vi "GetSourceAutorange.vi"(7 "SMU":T2, 8 "Error In":errorcluster, 10 "Source Function":T1, 11 "Kiethley 2602 In":refnum<visa-resource-name>) -> (0 "Error Out":errorcluster, 2 "Enabled?":bool, 3 "Keithley 2602 Out":refnum<visa-resource-name>)   [LabVIEW 2012, in "Keithley-2602.lvlib"]
uses:
  Keithley-2602.lvlib
  Controls/SMU.ctl
  Controls/SourceFunction.ctl
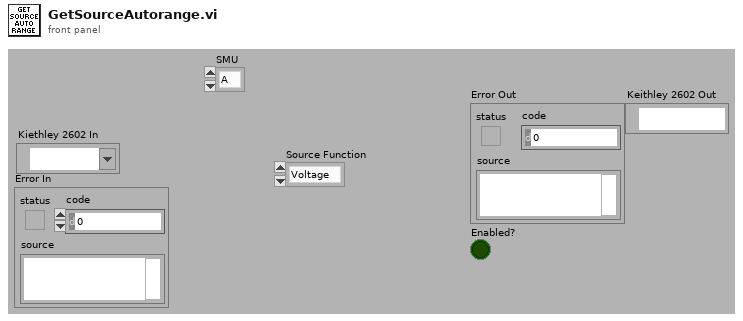
[diagram p1: front panel]
types:
  T1 = typedef "Keithley-2602.lvlib/SourceFunction.ctl" = enum16{"Voltage", "Current"}
  T2 = typedef "Keithley-2602.lvlib/SMU.ctl" = enum16{"A", "B"}
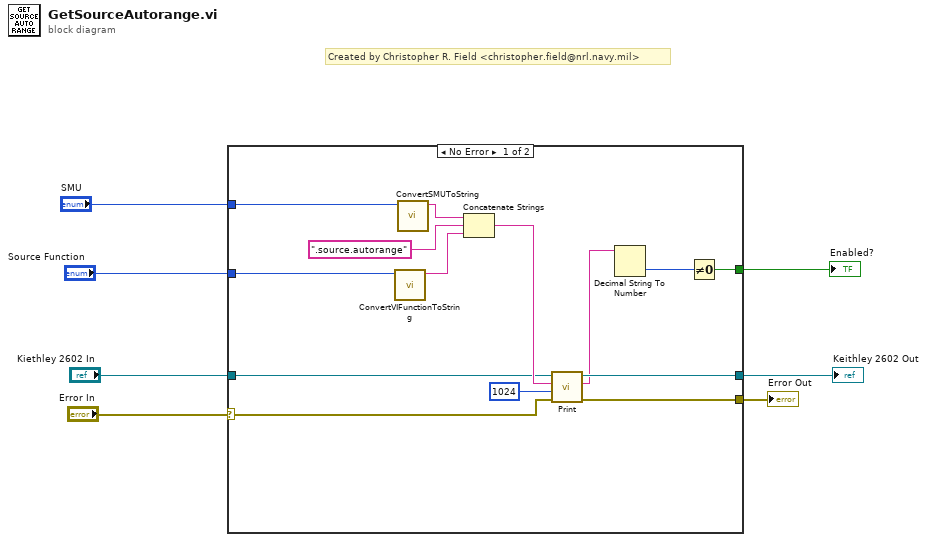
[diagram p0: block diagram]
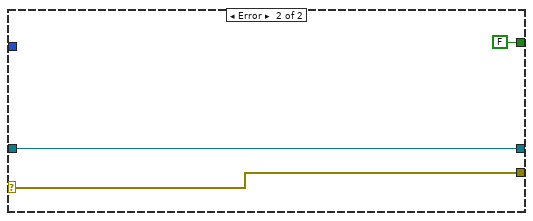
[diagram p2: hidden frame]
diagram:
  # "Created by Christopher R. Field <christopher.field@nrl.navy.mil>"
  n1 = case shown="No Error" "Error In" {
    selector: "Error In" -> [w8 w24]
    tunnel: "Kiethley 2602 In" -> [w17 w23]
    tunnel: [w16 w24] -> w6
    tunnel: [w15 w23] -> w5
    tunnel: [w12 FALSE] -> w4
    tunnel: "SMU" -> [w10 _]
    tunnel: "Source Function" -> [w9 _]
    frame No Error {
      n2 = call "ConvertVIFunctionToString.vi"("Function"=w9) -> ("Function (v or i)"=w11:string)  [unwired: 10 in]
      n3 = call "ConvertSMUToString.vi"("SMU"=w10) -> ("Channel"=w21:string)  [unwired: 10 in]
      n4 = Concatenate Strings(w21, ".source.autorange", w11) -> (w19:string)
      n5 = call "Print.vi"("Error In"=w8, "Byte Count"=u32 1024, "Attribute"=w19, "Kiethley 2602 In"=w17) -> ("Error Out"=w16:errorcluster, "Output"=w14:string, "Keithley 2602 Out"=w15:refnum<visa-resource-name>)  [unwired: 5 in]
      n6 = Decimal String To Number(string=w14) -> (number=w13:i32)  [unwired: 2 in, 1 out]
      n7 = Not Equal To 0?(x=w13) -> (x != 0?=w12:bool)
    }
    frame Error {
    }
  }
  "Error Out" <- w6
  "Keithley 2602 Out" <- w5
  "Enabled?" <- w4
